vi "New Humidity Test.vi"() -> ()   [LabVIEW 2012]
uses:
  Reusable/General/Temperature/Temperature.lvlib
  Devices/Alicat/Data/MC/AlicatMCData.lvclass
  Reusable/General/Atmospheric/Atmospheric Library.lvlib
  <vilib>/Utility/file.llb/Write To Spreadsheet File (DBL).vi
  <vilib>/Utility/file.llb/Write To Spreadsheet File (string).vi
  Reusable/Data/Data.lvclass
panel:
  out "Qdata":cluster{"Q":sgl, "P":sgl, "Q":sgl, "P":sgl}(graph)
  in  "Write?":bool
  out "RH_sat_calc":dbl
  in  "RH_sat_out":dbl caption="RHsat (%)"
  in  "Override":bool
  in  "MFC SP":sgl[](array[numeric])=[0.16, 0.0, 0.0, 0.0, 3.0, 0.0, 0.0, 0.0, 0.0, 0.0]
  out "Time":timestamp=timestamp(3396896939.1058674 s since 1904-01-01) format="%<%H:%M:%S%2u>T"
  in  "RHtarget":dbl=90.0 caption="RH (%)"
  in  "Vtec":dbl=1.6720317570902745 caption="TEC Voltage" min=0.0 max=6.0 step=0.01
  out "tecData":cluster{dbl, "Vtec":dbl, dbl}(graph)
  out "data":T1(graph)
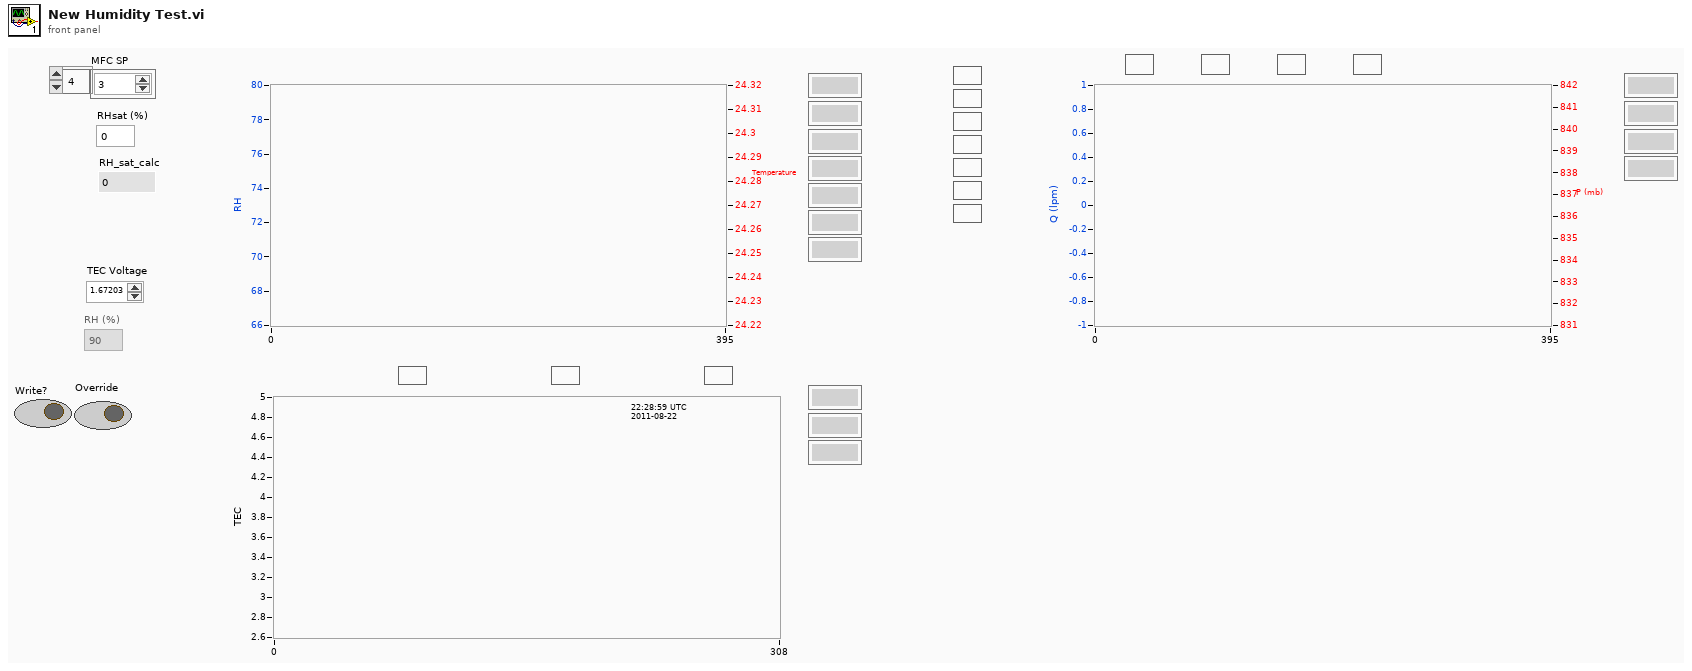
[diagram p1: front panel]
types:
  T1 = cluster{"[0]":dbl, "[1]":dbl, "[2]":dbl, "[3]":dbl, "[4]":dbl, "[5]":dbl, "[6]":dbl}
  T2 = enum8{"Enabled", "Disabled", "Disabled and Grayed Out"}
  T3 = cluster{"P":sgl, "T":sgl, "Q":sgl, "Q0":sgl, "Qsp":sgl}
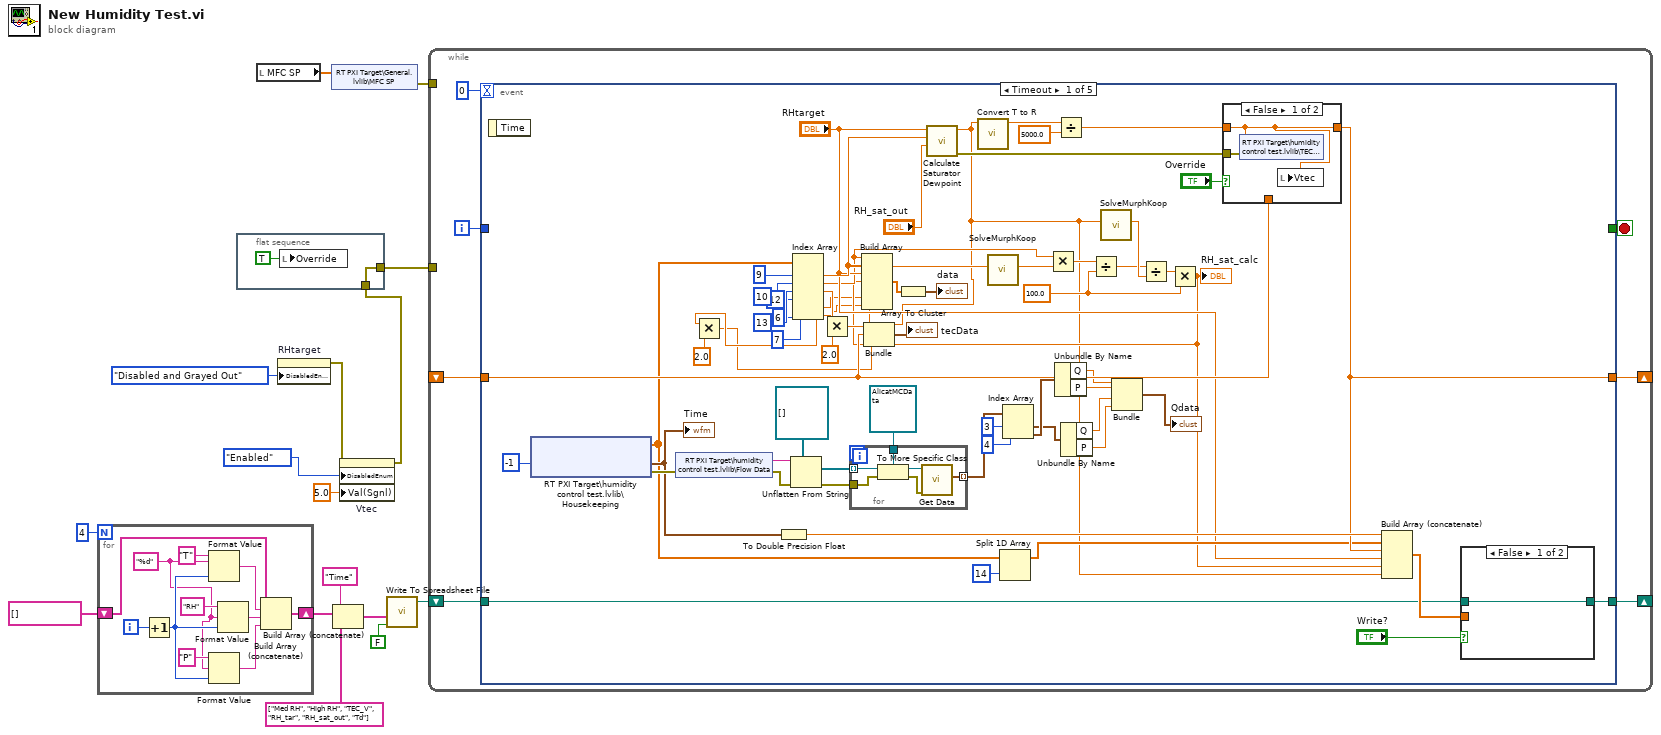
[diagram p0: block diagram]
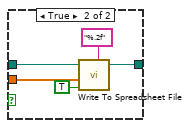
[diagram p2: hidden frame]
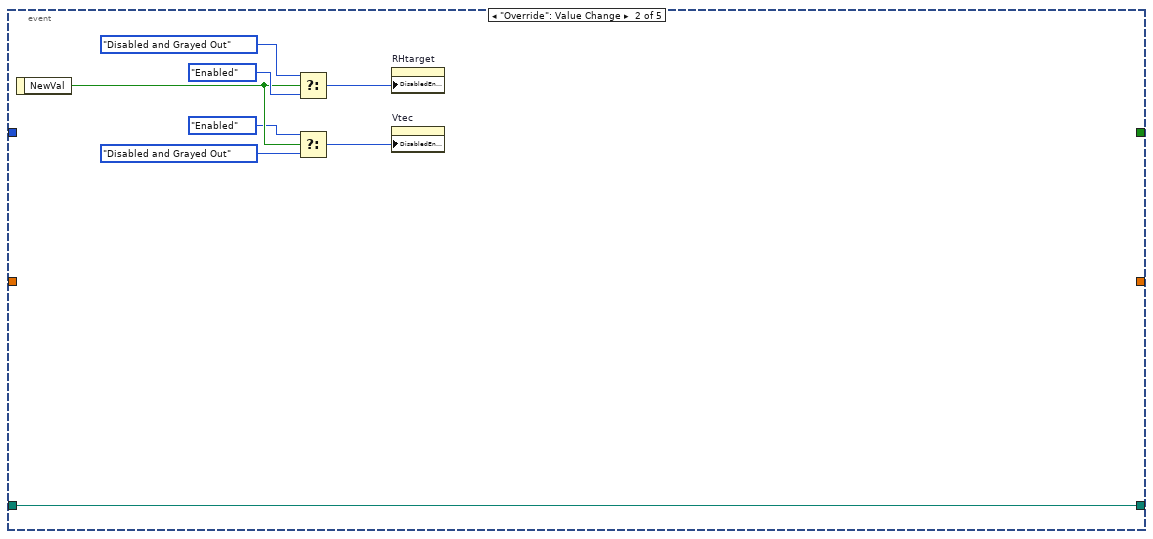
[diagram p4: hidden frame]
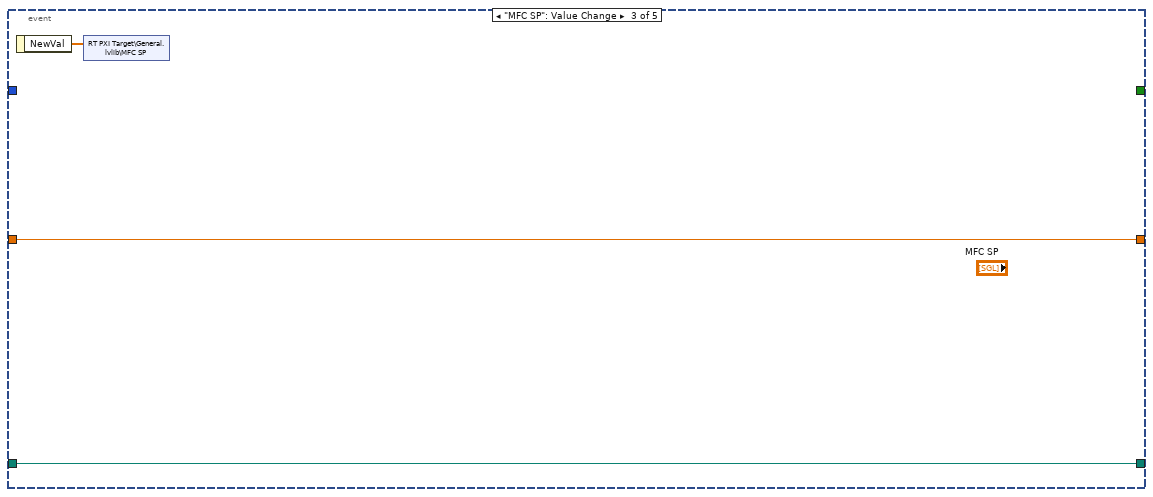
[diagram p5: hidden frame]
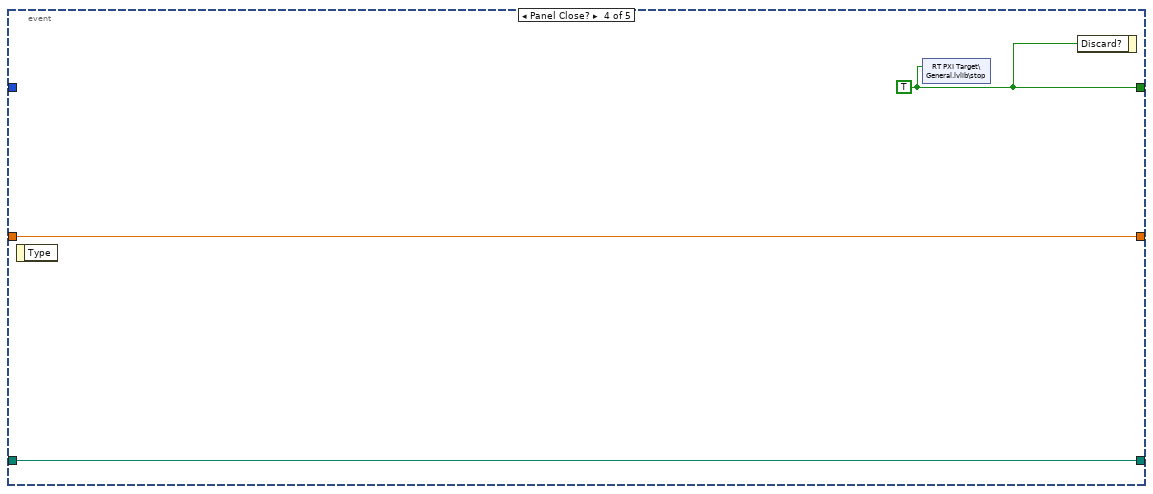
[diagram p6: hidden frame]
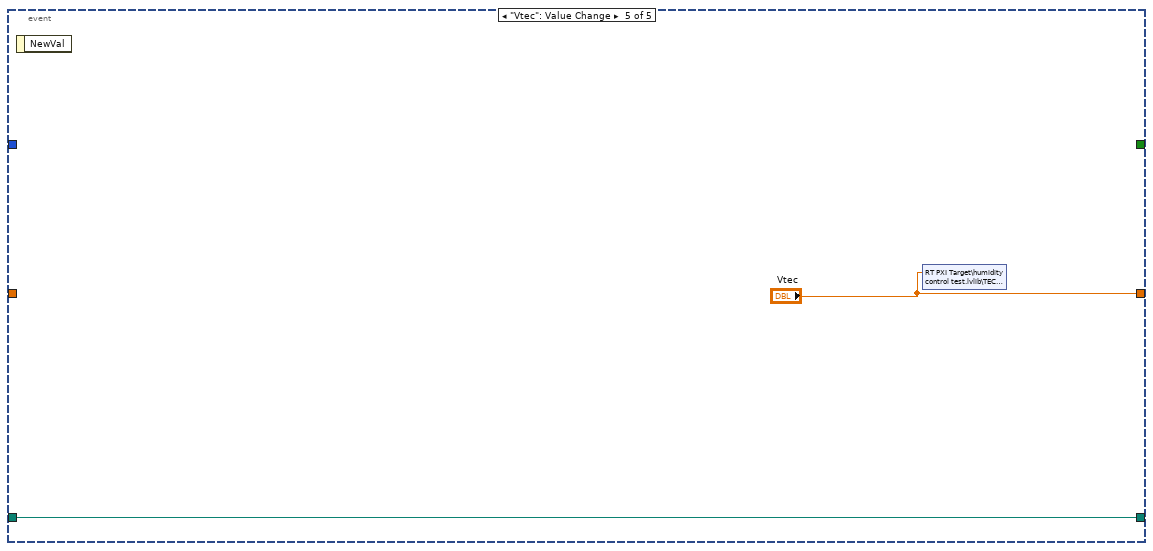
[diagram p7: hidden frame]
diagram:
  n1 = for {
    N: 4 -> [_]
    shift-right: [w19] -> w12
    shift-left: string[] [] -> [w18]
    i -> [w27]
    w17 = "%d" ("format string")
    n2 = Increment(x=w27) -> (x+1=w26:i32)
    n3 = Format Value(string ("")="T", format string=w17, value (0)=w26) -> (output string=w22:string)
    n4 = Format Value(string ("")="P", format string=w17, value (0)=w26) -> (output string=w20:string)
    n5 = Format Value(string ("")="RH", format string=w17, value (0)=w26) -> (output string=w21:string)
    n6 = Build Array (concatenate)(w18, w22, w21, w20) -> (w19:string[])
  }
  n7 = flat-sequence {
    tunnel: w3 -> [w28]
    tunnel: [w28] -> w2
    frame #0 {
      n8 = local write "Override"(TRUE ("Override")) -> ()
    }
  }
  n9 = local read "MFC SP"() -> (w16:sgl[])
  n10 = property on="RHtarget" class="DigNum (strict)"("DisabledEnum"=T2."Disabled and Grayed Out" ("Disabled")) -> (error out=w4:errorcluster)  [unwired: 2 in, 1 out]
  n11 = shared-variable "RT PXI Target\\General.lvlib\\MFC SP"(w16) -> (error out=w15:errorcluster)  [unwired: 1 in]
  n12 = Build Array (concatenate)("Time", w12, string[] ["Med RH", "High RH", "TEC_V", "RH_tar", "RH_sat_out", "Td"]) -> (w8:string[])
  n13 = property on="Vtec" class="DigNum (strict)"(error in=w4, "DisabledEnum"=T2."Enabled" ("Disabled"), "Val(Sgnl)"=5.0 ("Value (Signaling)")) -> (error out=w3:errorcluster)  [unwired: 1 in, 1 out]
  n14 = call-poly <vilib>:"Write To Spreadsheet File.vi"("append to file? (new file:F)"=FALSE, "1D data"=w8) -> ("new file path (Not A Path if cancelled)"=w9:path)  [unwired: 6 in]
  n15 = while {
    shift-right: [w33] -> _
    shift-left: _ -> [w32]
    tunnel: w15 -> [_]
    shift-right: [w31] -> _
    shift-left: w9 -> [w30]
    tunnel: w2 -> [_]
    i -> [w34]
    stop <- w36 stop-if-true
    n16 = event shown="[0] Timeout" {
      selector: _ -> [_ _ _ _ _]
      dyn-events: _ -> [_ _ _ _ _]
      timeout: 0 -> [_ _ _ _ _]
      tunnel: [_ _ _ w128 _] -> w36
      tunnel: w34 -> [_ _ _ _ _]
      tunnel: [w66 _ w125 w127 "Vtec"] -> w33
      tunnel: w32 -> [w69 _ w125 w127 _]
      tunnel: [w63 w115 w123 w126 w129] -> w31
      tunnel: w30 -> [w62 w115 w123 w126 w129]
      event Timeout {
        w77 = 100.0 ("y")
        n17 = event-data() -> ()  [unwired: 1 in, 1 out]
        n18 = shared-variable "RT PXI Target\\humidity control test.lvlib\\Housekeeping"(-1 ("ms timeout (0)")) -> (w61:dbl[], error out=w93:errorcluster, w68:timestamp)  [unwired: 1 in, 1 out]
        "Time" <- w68
        n19 = shared-variable "RT PXI Target\\humidity control test.lvlib\\Flow Data"(error in=w93) -> (w92:string, error out=w91:errorcluster)
        n20 = To Double Precision Float(number=w68) -> (double precision float=w67:dbl)
        n21 = Unflatten From String(type=refnum<class "Data.lvclass">[] [], binary string=w92, error in (no error)=w91) -> (value=w89:refnum<class "Data.lvclass">[], error out=w88:errorcluster)  [unwired: 2 in, 1 out]
        n22 = Index Array(array=w61, index #1=9 ("index"), index #2=10 ("index"), index #3=13 ("index"), index #4=12 ("index"), index #5=6 ("index"), index #6=7 ("index")) -> (element #1=w73:dbl, element #2=w57:dbl, element #3=w75:dbl, element #4=w44:dbl, element #5=w40:dbl, element #6=w39:dbl)
        n23 = Multiply(x=w44, y=2.0 ("x")) -> (x*y=w43:dbl)
        n24 = Multiply(x=w75, y=2.0 ("x")) -> (x*y=w84:dbl)
        n25 = for {
          tunnel: w89 -> [w114] mode=indexing
          tunnel: w88 -> [w113]
          tunnel: refnum<class "AlicatMCData.lvclass"> refnum ("Alicat.lvlib:AlicatMCData.lvclass") -> [w112]
          tunnel: [w109] -> w54 mode=indexing
          n26 = To More Specific Class(target class=w112, reference=w114, error in=w113) -> (specific class reference=w111:refnum<class "AlicatMCData.lvclass">, error out=w110:errorcluster)
          n27 = call "Get Data.vi"("error in"=w110, "AlicatMData in"=w111) -> ("SystemData"=w109:T3)  [unwired: 7 in, 2 out]
        }
        n28 = Bundle(w84, "Vtec"=w69, w43) -> (→"tecData":cluster{dbl, "Vtec":dbl, dbl})  [unwired: 1 in]
        n29 = call "Calculate Saturator Dewpoint.vi"("RH_sat_out"="RH_sat_out", "Tair"=w73, "RH_tar"="RHtarget") -> ("error out"=w82:errorcluster, "Td"=w55:dbl)  [unwired: 7 in]
        n30 = call "Convert T to R.vi"("T"=w55) -> ("R"=w86:dbl)  [unwired: 10 in]
        n31 = call "SolveMurphKoop.vi"("T"=w73) -> ("es"=w72:dbl)  [unwired: 7 in, 3 out]
        n32 = Split 1D Array(array=w61, index=14) -> (first subarray=w59:dbl[])  [unwired: 1 out]
        n33 = Index Array(array=w54, index #1=3 ("index"), index #2=4 ("index")) -> (element #1=w37:T3, element #2=w38:T3)
        n34 = Multiply(x=w57, y=w72) -> (x*y=w81:dbl)
        n35 = Unbundle By Name(w38) -> ("Q"=w51:sgl, "P"=w50:sgl)
        n36 = Divide(x=w86, y=5000.0) -> (x/y=w71:dbl)
        n37 = Unbundle By Name(w37) -> ("Q"=w49:sgl, "P"=w48:sgl)
        n38 = Divide(x=w81, y=w77) -> (x/y=w79:dbl)
        n39 = call "SolveMurphKoop.vi"("T"=w55) -> ("es"=w80:dbl)  [unwired: 7 in, 3 out]
        n40 = Bundle("Q"=w51, "P"=w50, "Q"=w49, "P"=w48) -> (→"Qdata":cluster{"Q":sgl, "P":sgl, "Q":sgl, "P":sgl})  [unwired: 1 in]
        n41 = Divide(x=w79, y=w80) -> (x/y=w78:dbl)
        n42 = Multiply(x=w78, y=w77) -> (x*y=w56:dbl)
        "RH_sat_calc" <- w56
        n43 = Build Array(w57, w73, "RHtarget", w56, w55, w40, w39) -> (w97:dbl[])
        n44 = Array To Cluster(array=w97) -> (cluster=→"data":T1)
        n45 = case shown="False" "Override" {
          tunnel: w82 -> [w107 _]
          tunnel: w71 -> [w106 _]
          tunnel: [w106 w108] -> w66
          tunnel: w69 -> [_ w108]
          frame False {
            n46 = shared-variable "RT PXI Target\\humidity control test.lvlib\\TEC_SP"(w106, error in=w107) -> ()  [unwired: 1 out]
            n47 = local write "Vtec"(w106) -> ()
          }
          frame True {
          }
        }
        n48 = Build Array (concatenate)(w67, w59, w66, "RHtarget", w56, w55) -> (w64:dbl[])
        n49 = case shown="False" "Write?" {
          tunnel: w64 -> [_ w105]
          tunnel: [w100 w103] -> w63
          tunnel: w62 -> [w100 w102]
          frame False {
          }
          frame True {
            n50 = call-poly <vilib>:"Write To Spreadsheet File.vi"("format (%.3f)"="%.2f", "append to file? (new file:F)"=TRUE, "1D data"=w105, "file path (dialog if empty)"=w102) -> ("new file path (Not A Path if cancelled)"=w103:path)  [unwired: 4 in]
          }
        }
      }
      event "Override": Value Change {
        n51 = event-data() -> ("NewVal"=w120:bool)  [unwired: 1 in]
        n52 = Select(t=T2."Disabled and Grayed Out", s=w120, f=T2."Enabled" ("Disabled")) -> (s? t:f=w117:T2)
        n53 = Select(t=T2."Enabled" ("Disabled"), s=w120, f=T2."Disabled and Grayed Out" ("t")) -> (s? t:f=w116:T2)
        n54 = property on="RHtarget" class="DigNum (strict)"("DisabledEnum"=w117) -> ()  [unwired: 2 in, 2 out]
        n55 = property on="Vtec" class="DigNum (strict)"("DisabledEnum"=w116) -> ()  [unwired: 2 in, 2 out]
      }
      event "MFC SP": Value Change {
        n56 = event-data() -> ("NewVal"=w124:sgl[])  [unwired: 1 in]
        n57 = shared-variable "RT PXI Target\\General.lvlib\\MFC SP"(w124) -> ()  [unwired: 1 in, 1 out]
      }
      event Panel Close? {
        w128 = TRUE ("Discard?")
        n58 = event-data() -> ()  [unwired: 1 in, 1 out]
        n59 = shared-variable "RT PXI Target\\General.lvlib\\stop"(w128) -> ()  [unwired: 1 in, 1 out]
        n60 = event-data("Discard?"=w128) -> ()  [unwired: 1 in, 1 out]
      }
      event "Vtec": Value Change {
        n61 = event-data() -> ()  [unwired: 1 in, 1 out]
        n62 = shared-variable "RT PXI Target\\humidity control test.lvlib\\TEC_SP"("Vtec") -> ()  [unwired: 1 in, 1 out]
      }
    }
  }
